vi "MotionProfileController.vi"(0 "Target Pos":dbl, 1 "MaxVel":dbl=80.0, 2 "MaxAccel":dbl=150.0, 5 "Robot":cluster{"Pos":dbl, "Vel":dbl}={"Pos"=26.0882735, "Vel"=0.0}, 7 "Gains":T1={"Gains"={"FFV"=0.0061, "FFA"=0.0024, "Vel PID"={"P"=0.0, "I"=0.0, "D"=0.0}}, "Pos PID"={"P"=0.0, "I"=0.0, "D"=0.0}} {"Pos PID"."D" format="%.3f"; "Pos PID"."I" format="%.3f"; "Pos PID"."P" format="%.3f"; "Gains"."Vel PID"."D" format="%.3f"; "Gains"."Vel PID"."I" format="%.3f"; "Gains"."Vel PID"."P" format="%.3f"}, 9 "Delay":dbl=20.0, 11 "Reset":bool) -> (4 "Power":dbl(graph)=0.25, 8 "Distance":cluster{"Output":dbl, "dx/dt":dbl}(graph)={"Output"=52.36486996421861, "dx/dt"=26.0882735}, 10 "Done":bool, 15 "VelGraph":cluster{"Output":dbl, "dx/dt":dbl}(graph))   [LabVIEW 2018]
uses:
  <vilib>/addons/control/pid/pid.llb/PID (DBL).vi
  <vilib>/addons/control/pid/NI_PID_pid.lvlib
panel:
  in  "Target Vel":dbl
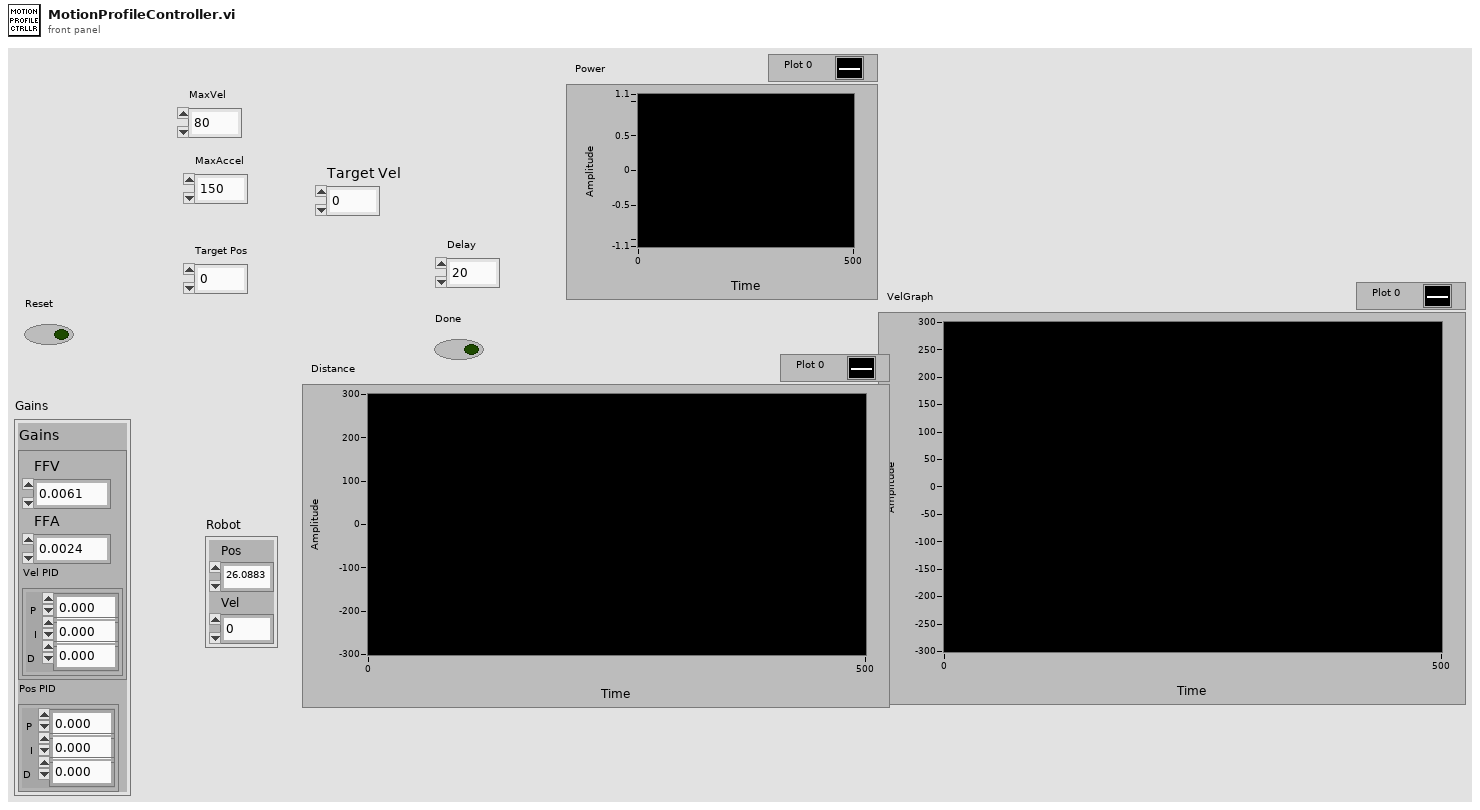
[diagram p1: front panel]
types:
  T1 = cluster{"Gains":cluster{"FFV":dbl, "FFA":dbl, "Vel PID":cluster{"P":dbl, "I":dbl, "D":dbl}}, "Pos PID":cluster{"P":dbl, "I":dbl, "D":dbl}}
  T2 = cluster{"TargetPos":dbl, "InitalPos":dbl, "FinalVel":dbl, "IntitialVel":dbl, "MaxVel":dbl, "MaxAccel":dbl}
  T3 = cluster{"FFV":dbl, "FFA":dbl, "Vel PID":cluster{"P":dbl, "I":dbl, "D":dbl}}
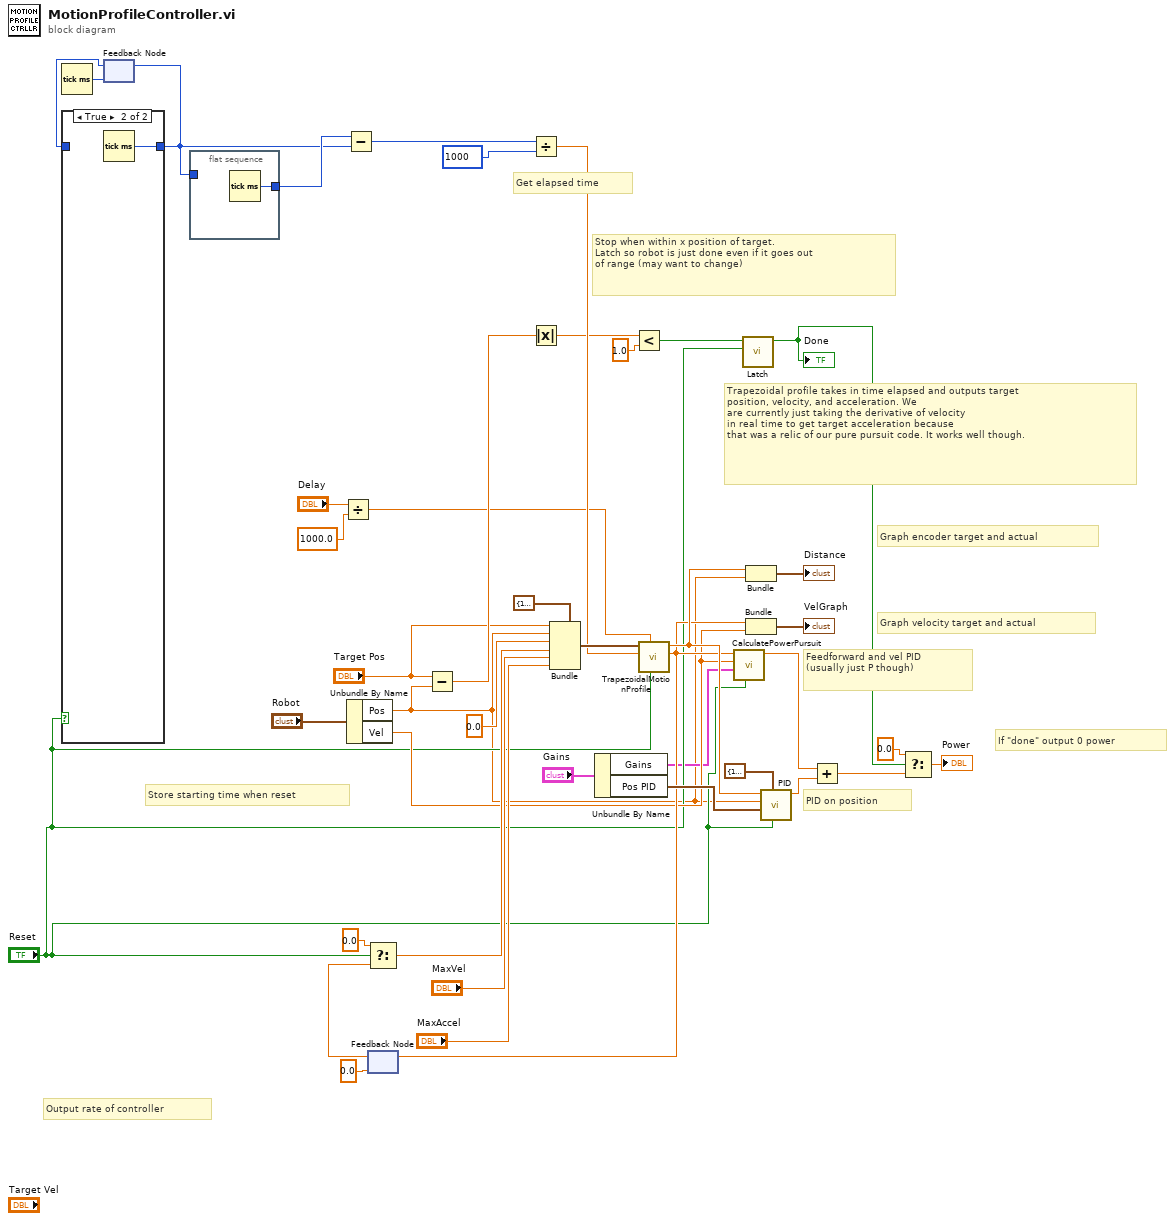
[diagram p0: block diagram]
diagram:
  # "Output rate of controller"
  # "If \"done\" output 0 power"
  # "Graph velocity target and actual"
  # "Graph encoder target and actual"
  # "Feedforward and vel PID\n(usually just P though)"
  # "Trapezoidal profile takes in time elapsed and outputs target\nposition, velocity, and acceleration. We\nare currently just taking the derivative of velocity\nin real time to get target acceleration because\nthat was a relic of our pure pursuit code. It works well though."
  # "PID on position"
  # "Get elapsed time"
  # "Store starting time when reset"
  # "Stop when within x position of target.\nLatch so robot is just done even if it goes out\nof range (may want to change)"
  n1 = Tick Count (ms)() -> (millisecond timer value=w22:u32)
  n2 = feedback #1(w22) -> (w23:u32)
  n3 = case shown="True" "Reset" {
    tunnel: [w43 w44] -> w17
    tunnel: w23 -> [w43 _]
    frame False {
    }
    frame True {
      n4 = Tick Count (ms)() -> (millisecond timer value=w44:u32)
    }
  }
  n5 = feedback-in #1(w17) -> ()
  n6 = flat-sequence {
    tunnel: [w45] -> w37
    tunnel: w17 -> [_]
    frame #0 {
      n7 = Tick Count (ms)() -> (millisecond timer value=w45:u32)
    }
  }
  n8 = Divide(x="Delay", y=1000.0) -> (x/y=w1:dbl)
  n9 = Subtract(x=w37, y=w17) -> (x-y=w36:u32)
  n10 = Unbundle By Name("Robot") -> ("Pos"=w6:dbl, "Vel"=w10:dbl)
  n11 = feedback #2(0.0 ("Velocity")) -> (w11:dbl)
  n12 = Select(t=0.0, s="Reset", f=w11) -> (s? t:f=w14:dbl)
  n13 = Subtract(x="Target Pos", y=w6) -> (x-y=w5:dbl)
  n14 = Divide(x=w36, y=u32 1000) -> (x/y=w34:dbl)
  n15 = Absolute Value(x=w5) -> (abs(x)=w19:dbl)
  n16 = Bundle(cluster=T2 {"TargetPos"=10.0, "InitalPos"=0.0, "FinalVel"=0.0, "IntitialVel"=0.0, "MaxVel"=10.0, "MaxAccel"=10.0} ("Config"), "TargetPos"="Target Pos", "InitalPos"=w6, "FinalVel"=0.0 ("IntitialVel"), "IntitialVel"=w14, "MaxVel"="MaxVel", "MaxAccel"="MaxAccel") -> (w38:T2)
  n17 = Unbundle By Name("Gains") -> ("Gains"=w7:T3, "Pos PID"=w27:cluster{"P":dbl, "I":dbl, "D":dbl})
  n18 = Less?(x=w19, y=1.0) -> (x < y?=w30:bool)
  n19 = call "TrapezoidalMotionProfile.vi"("Initialize"="Reset", "dt"=w1, "Time"=w34, "Config"=w38) -> ("Velocity"=w13:dbl, "Distance"=w25:dbl)  [unwired: 4 in, 2 out]
  n20 = feedback-in #2(w13) -> ()
  n21 = call "CalculatePowerPursuit.vi"("Reset"="Reset", "Gains"=w7, "Vel"=w10, "Target Vel"=w13) -> ("Power"=w20:dbl)  [unwired: 7 in]
  n22 = call "Latch.vi"("Reset"="Reset", "Input"=w30) -> ("Output"=w15:bool)  [unwired: 9 in]
  "Done" <- w15
  n23 = Bundle("Distance"=w25, "Pos"=w6) -> (→"Distance":cluster{"Distance":dbl, "Pos":dbl})  [unwired: 1 in]
  n24 = Bundle("Velocity"=w13, "Vel"=w10) -> (→"VelGraph":cluster{"Velocity":dbl, "Vel":dbl})  [unwired: 1 in]
  n25 = call-poly <vilib>:"PID.vi"("reinitialize? (F)"="Reset", "output range"=cluster{"output high":dbl, "output low":dbl} {"output high"=1.0, "output low"=-1.0}, "PID gains"=w27, "process variable"=w6, "setpoint"=w25) -> ("output"=w21:dbl)  [unwired: 5 in, 1 out]
  n26 = Add(x=w20, y=w21) -> (x+y=w16:dbl)
  n27 = Select(t=0.0, s=w15, f=w16) -> (s? t:f=→"Power":dbl)
